vi "De-Initialize.vi"(8 "error in (no error)":errorcluster, 11 "Quantum Design Driver in":refnum<class "Quantum Design Driver.lvclass">) -> (0 "error out":errorcluster, 3 "Quantum Design Driver out":refnum<class "Quantum Design Driver.lvclass">)   [LabVIEW 2021, in "Quantum Design Driver.lvclass"]
uses:
  Quantum Design Driver.lvclass
  Quantum Design Driver.lvclass/Quantum Design Driver.ctl
  Simple VISA Reader/Simple VISA Reader Driver.lvclass
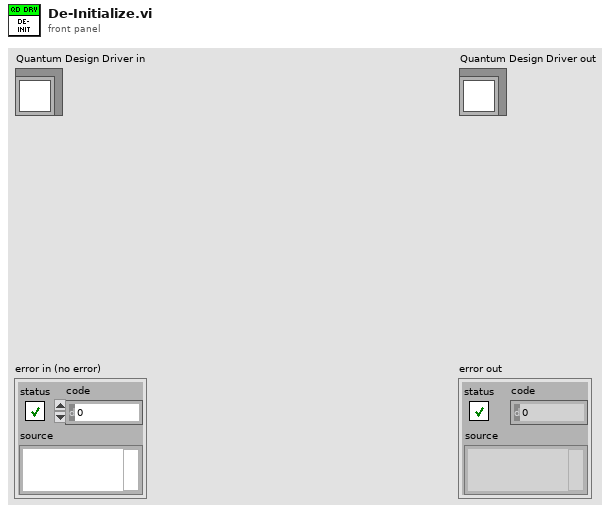
[diagram p1: front panel]
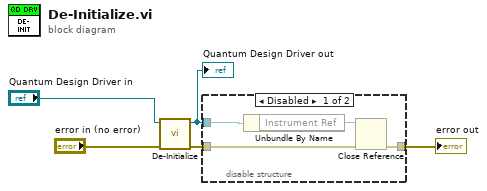
[diagram p0: block diagram]
diagram:
  n1 = call-parent "De-Initialize.vi"("error in (no error)"="error in (no error)", "Instrument Driver in"="Quantum Design Driver in") -> ("error out"=w2:errorcluster, "Instrument Driver out"=w3:refnum<class "Quantum Design Driver.lvclass">)  [unwired: 8 in]
  "Quantum Design Driver out" <- w3
  n2 = disable-structure shown="Disabled" {
    disable-tunnel: w3 -> [w9 _]
    disable-tunnel: w2 -> [w7 w10]
    disable-tunnel: [w6 w10] -> w1
    frame Disabled {
      n3 = Unbundle By Name(w9) -> ("Instrument Ref"=w8:refnum<k24>)
      n4 = Close Reference(reference=w8, error in (no error)=w7) -> (error out=w6:errorcluster)
    }
    frame Enabled {
    }
  }
  "error out" <- w1
